vi "Send New Test Record.vi"(8 "error in":errorcluster, 11 "Stim Player Data In":T1) -> (0 "error out":errorcluster, 3 "Stim Player Data Out":T1)   [LabVIEW 2011]
uses:
  Controls/Stim Player Data.ctl
  Controls/Top Level Control.ctl
  <vilib>/NI/AMC/Message Queue.ctl
  <vilib>/NI/AMC/Message.ctl
  <vilib>/NI/Tools/Keyed Array/KeyedArray.ctl
  Controls/ListBox Test Record.ctl
  Controls/DVR of CSV Tests Data.ctl
  Controls/CSVs Tests Data.ctl
  Controls/Test Column Data.ctl
  Controls/Options DVR.ctl
  Controls/Options.ctl
  <vilib>/NI Veristand/Execution/Workspace/WorkspaceAPI.ctl
  NationalInstruments.VeriStand.ClientAPI
  <vilib>/NI Veristand/Execution/SequenceExecutionInterface/Stimulus Profile Session Ref.ctl
  <vilib>/NI Veristand/Execution/ChannelFaultManager/ChannelFaultAPI.ctl
  <vilib>/NI/AMC/Create Single Message.vi
  <vilib>/NI/AMC/Update Message Routing Info.vi
  <vilib>/NI/AMC/Send Message.vi
  <vilib>/NI/AMC/AMC.lvlib
  <vilib>/NI/Tools/Keyed Array/Tools_KeyedArray.lvlib
  <vilib>/NI Veristand/Execution/Workspace/NI_VS Workspace ExecutionAPI.lvlib
  <vilib>/NI Veristand/Execution/SequenceExecutionInterface/NI_VS Sequence Execution Interface.lvlib
  <vilib>/NI Veristand/Execution/ChannelFaultManager/NI_VS ChannelFault ExecutionAPI.lvlib
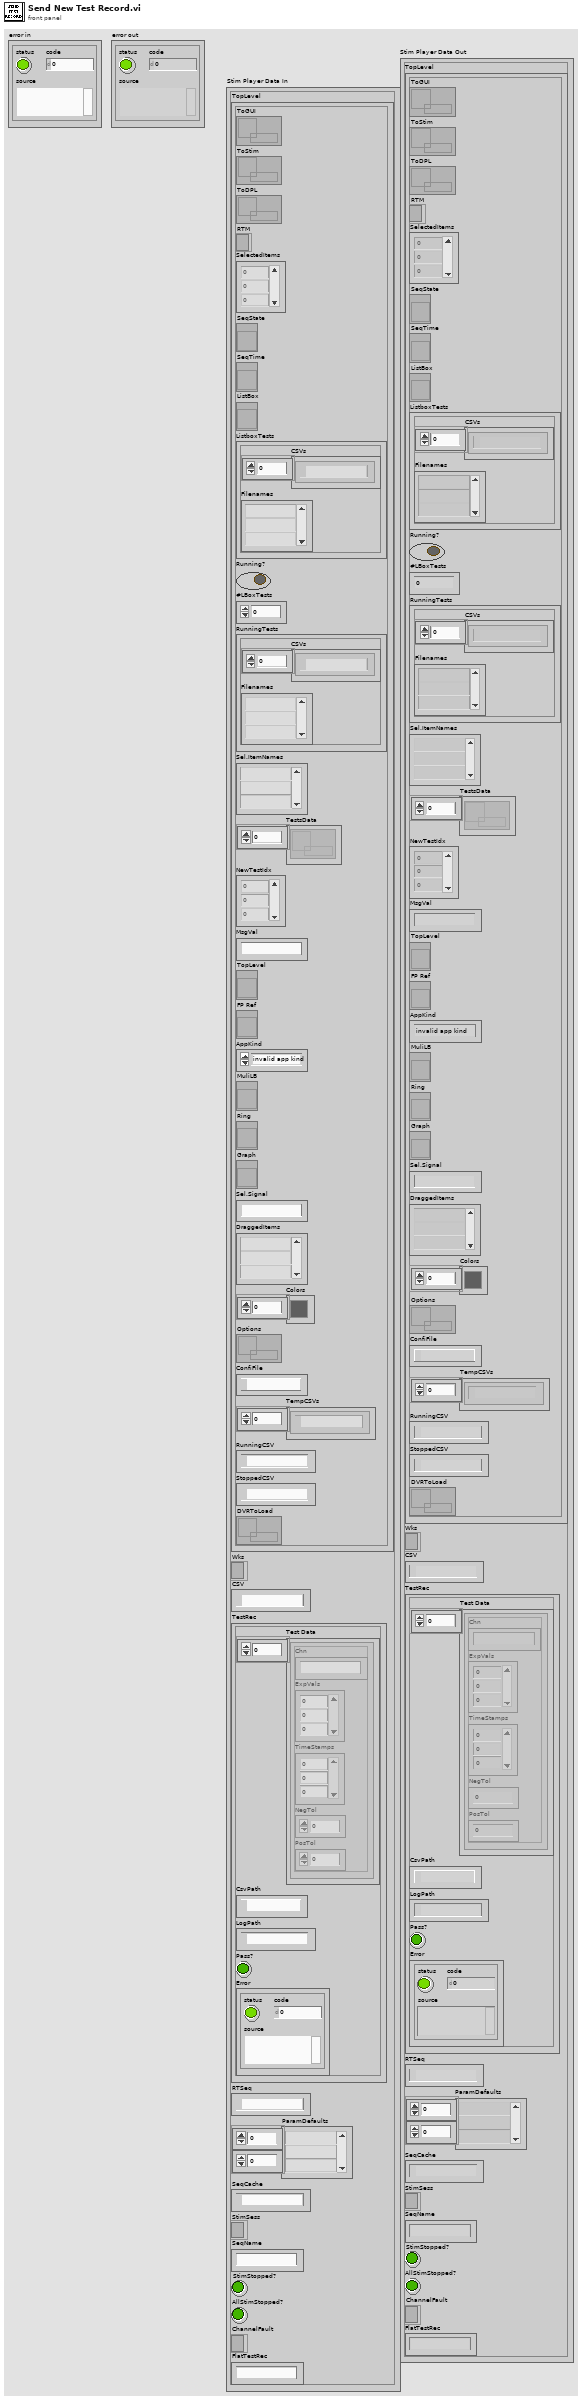
[diagram p1: front panel]
types:
  T1 = typedef "Stim Player Data.ctl" = cluster{"TopLevel":T2, "Wks":T7, "CSV":path, "TestRec":T8, "RTSeq":path, "ParamDefaults":string[][], "SeqCache":path, "StimSess":T10, "SeqName":string, "StimStopped?":bool, "AllStimStopped?":bool, "ChannelFault":T11, "FlatTestRec":string}
  T2 = typedef "Top Level Control.ctl" = cluster{"ToGUI":T3, "ToStim":T3, "ToDPL":T3, "RTM":refnum<k9>, "SelectedItems":i32[], "SeqState":refnum<vi>, "SeqTime":refnum<vi>, "ListBox":refnum<vi>, "ListboxTests":T4, "Running?":bool, "#LBoxTests":i32, "RunningTests":T4, "Sel.ItemNames":string[], "TestsData":T5[], "NewTestIdx":i32[], "MsgVal":string, "TopLevel":refnum<vi>, "FP Ref":refnum<vi>, "AppKind":enum32{"invalid app kind", "Development System", "Run Time System", "Student Edition", "Embedded LabVIEW", "Evaluation", "Custom"}, "MuliLB":refnum<vi>, "Ring":refnum<vi>, "Graph":refnum<vi>, "Sel.Signal":string, "DraggedItems":string[], "Colors":u32[], "Options":T6, "ConfiFile":path, "TempCSVs":path[], "RunningCSV":path, "StoppedCSV":path, "DVRToLoad":T5}
  T3 = typedef "AMC.lvlib/Message Queue.ctl" = refnum<queue>
  T4 = typedef "ListBox Test Record.ctl" = cluster{"CSVs":path[], "Filenames":string[]}
  T5 = typedef "DVR of CSV Tests Data.ctl" = refnum<data-value>
  T6 = typedef "Options DVR.ctl" = refnum<data-value>
  T7 = typedef "NI_VS Workspace ExecutionAPI.lvlib/WorkspaceAPI.ctl" = refnum<k24>
  T8 = typedef "CSVs Tests Data.ctl" = cluster{"Test Data":T9[], "CsvPath":path, "LogPath":path, "Pass?":bool, "Error":errorcluster}
  T9 = typedef "Test Column Data.ctl" = cluster{"Chn":string, "ExpVals":dbl[], "TimeStamps":i64[], "NegTol":dbl, "PosTol":dbl}
  T10 = typedef "NI_VS Sequence Execution Interface.lvlib/Stimulus Profile Session Ref.ctl" = refnum<k24>
  T11 = typedef "NI_VS ChannelFault ExecutionAPI.lvlib/ChannelFaultAPI.ctl" = refnum<k24>
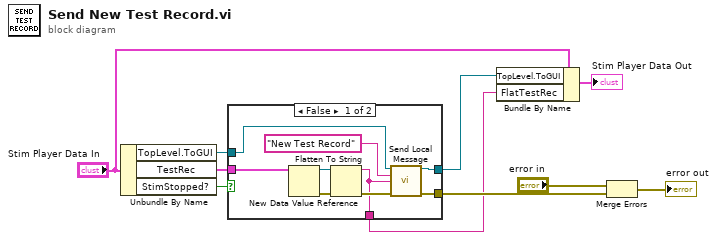
[diagram p0: block diagram]
diagram:
  n1 = Unbundle By Name("Stim Player Data In") -> ("TopLevel.ToGUI"=w5:T3, "TestRec"=w2:T8, "StimStopped?"=w3:bool)
  n2 = case shown="False" w3 {
    tunnel: [w16 _] -> w10
    tunnel: w5 -> [w14 w20]
    tunnel: [w13 w20] -> w4
    tunnel: w2 -> [w12 _]
    tunnel: [w11 _] -> w1
    frame False {
      n3 = New Data Value Reference(data value=w12) -> (data value reference=w18:refnum<data-value>, error out=w19:errorcluster)  [unwired: 1 in]
      n4 = Flatten To String(anything=w18, error in (no error)=w19) -> (data string=w11:string, error out=w17:errorcluster)  [unwired: 2 in, 1 out]
      n5 = call <vilib>:"Send Local Message.vi"("message queue in"=w14, "message name"="New Test Record" ("message"), "message value"=w11, "error in"=w17) -> ("message queue out"=w13:T3, "error out"=w16:errorcluster)  [unwired: 9 in, 1 out]
    }
    frame True {
    }
  }
  n6 = Bundle By Name(cluster="Stim Player Data In", "TopLevel.ToGUI"=w4, "FlatTestRec"=w1) -> (→"Stim Player Data Out":T1)
  n7 = Merge Errors("error in", w10) -> (→"error out":errorcluster)
